vi "Joystick to Turret Angle.vi"(8 "Deadband Upper":dbl, 9 "Deadband Lower":dbl, 10 "Y":dbl(slide) scale=1.0..-1.0, 11 "X":dbl(slide) scale=-1.0..1.0) -> (2 "In Range?":bool, 3 "Angle":dbl)   [LabVIEW 2019]
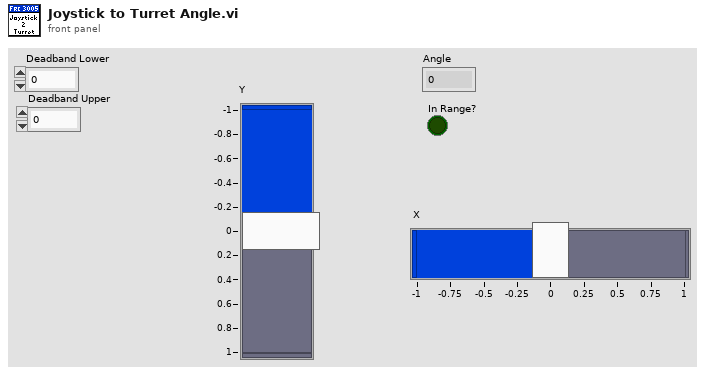
[diagram p1: front panel]
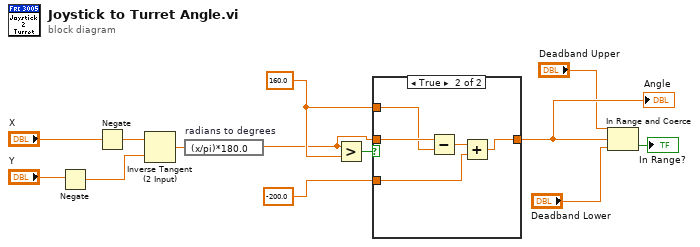
[diagram p0: block diagram]
diagram:
  w7 = 160.0 ("upper limit")
  n1 = Negate(x="Y") -> (-x=w9:dbl)
  n2 = Negate(x="X") -> (-x=w10:dbl)
  n3 = Inverse Tangent (2 Input)(1:w9, 2:w10) -> (0:w13:dbl)
  n4 = expression code="(x/pi)*180.0" "radians to degrees"(w13) -> (w5:dbl)
  n5 = Greater?(x=w5, y=w7) -> (0:w6:bool)
  n6 = case shown="True" w6 {
    tunnel: w5 -> [w14 w19]
    tunnel: [w14 w16] -> w4
    tunnel: w7 -> [_ w18]
    tunnel: -200.0 ("lower limit") -> [_ w15]
    frame False {
    }
    frame True {
      n7 = Subtract(x=w19, y=w18) -> (x-y=w17:dbl)
      n8 = Add(x=w17, y=w15) -> (x+y=w16:dbl)
    }
  }
  "Angle" <- w4
  n9 = In Range and Coerce(upper limit="Deadband Upper", x=w4, lower limit="Deadband Lower") -> (In Range?=→"In Range?":bool)  [unwired: 1 out]
